vi "数据库存.vi"(7 "位移输入":dbl[](array[numeric]), 8 "错误输入（无错误）":errorcluster, 9 "载荷输入":dbl[](array[numeric]), 10 "电量输入":dbl[](array[numeric]), 11 "自动化引用句柄输入":refnum<k7>) -> (0 "错误输出":errorcluster, 3 "自动化引用句柄输出":refnum<k7>)   [LabVIEW 2018]
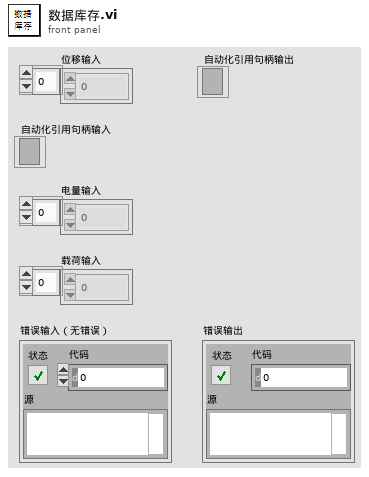
[diagram p1: front panel]
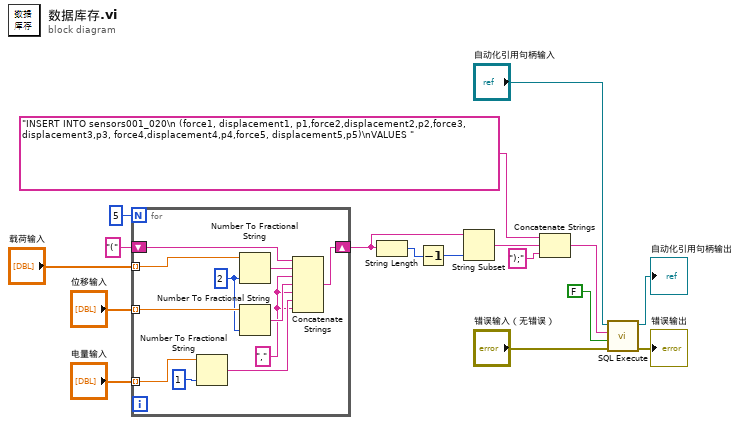
[diagram p0: block diagram]
diagram:
  n1 = for {
    N: 5 -> [_]
    tunnel: "载荷输入" -> [w27] mode=indexing
    tunnel: "位移输入" -> [w28] mode=indexing
    tunnel: "电量输入" -> [w23] mode=indexing
    shift-right: [w19] -> w12
    shift-left: "(" -> [w18]
    w26 = i16 2 ("宽度(-)")
    w20 = "," ("字符串")
    n2 = Number To Fractional String(number=w23, precision (6)=i16 1 ("精度(6)")) -> (F-format string=w21:string)  [unwired: 2 in]
    n3 = Number To Fractional String(number=w27, precision (6)=w26) -> (F-format string=w25:string)  [unwired: 2 in]
    n4 = Number To Fractional String(number=w28, precision (6)=w26) -> (F-format string=w24:string)  [unwired: 2 in]
    n5 = Concatenate Strings(w18, w25, w20, w24, w20, w21, w20) -> (w19:string)
  }
  n6 = String Length(string=w12) -> (length=w13:i32)
  n7 = Decrement(x=w13) -> (x-1=w14:i32)
  n8 = String Subset(string=w12, length (rest)=w14) -> (substring=w11:string)  [unwired: 1 in]
  n9 = Concatenate Strings("INSERT INTO sensors001_020\n (force1, displacement1, p1,force2,displacement2,p2,force3, displacement3,p3, force4,displacement4,p4,force5, displacement5,p5)\nVALUES " ("Command Text"), w11, ");") -> (w8:string)
  n10 = call <userlib>:"SQL Execute.vi"("error in (no error)"="错误输入（无错误）", "Return Data (T)"=FALSE, "Command Text"=w8, "ADODB._Connection In"="自动化引用句柄输入") -> ("error out"=→"错误输出":errorcluster, "ADODB._Connection Out"=→"自动化引用句柄输出":refnum<k7>)  [unwired: 4 in, 2 out]
